vi "cRIO_4DoF_InvYaw_global2mouse_v2.vi"(10 "op-space pos":dbl[](array[numeric]), 11 "op_vel":dbl[](array[numeric])) -> (3 "vel_out":dbl[](array[numeric]))   [LabVIEW 2019]
uses:
  <vilib>/imath/engines/lvmath2/RunTimeEngine/Managers/WorkSpace/UID Generator.vi
  <vilib>/imath/engines/lvmath2/RunTimeEngine/BuiltInFunctions/size/NIMS_[I32,I32]=size(GRow).vi
  <instcachedir>/0/NIMS_[I32,I32]=size(GRow)_CFE2C4BDC5BC45CD88F2F6A295A2273D.lvgen/NIMS_[I32,I32]=size(GRow)_CFE2C4BDC5BC45CD88F2F6A295A2273D_001.vi
  <vilib>/imath/engines/lvmath2/RunTimeEngine/RunTimeType/NIMS_RunTimeType_From StrictType (excl LVString).vi
  <instcachedir>/0/NIMS_RunTimeType_From StrictType (excl LVString)_D8AFBA86A94845AAA577C895450664BD.lvgen/NIMS_RunTimeType_From StrictType (excl LVString)_D8AFBA86A94845AAA577C895450664BD_000.vi
  <vilib>/imath/engines/lvmath2/RunTimeEngine/LocalVariableDefStatement/MC_LocalVariableDefStatement_Display.vi
  <vilib>/imath/engines/lvmath2/RunTimeEngine/IndexRead/NIMS M(R2,S).vi
  <instcachedir>/0/NIMS M(R2,S)_56813DCFDD5A484292D2195AF15D2BF5.lvgen/NIMS M(R2,S)_56813DCFDD5A484292D2195AF15D2BF5_000.vi
  <vilib>/imathl/engines/lvmath/Functions/Error Handling/Create Error.vi
  <vilib>/imath/engines/lvmath2/RunTimeEngine/ArithmeticOperatorToken/NIMS_ArithmeticOperator_multmx(M,CV)-internal.vi
  <instcachedir>/0/NIMS_ArithmeticOperator_multmx(M,CV)-internal_2C55777844884EEDB828A940D397C7D0.lvgen/NIMS_ArithmeticOperator_multmx(M,CV)-internal_2C55777844884EEDB828A940D397C7D0_001.vi
  <vilib>/imath/engines/lvmath2/RunTimeEngine/IndexRead/NIMS M(S,S).vi
  <instcachedir>/0/NIMS M(S,S)_AC51E74150A542F7991B9634C66F3096.lvgen/NIMS M(S,S)_AC51E74150A542F7991B9634C66F3096_000.vi
  <vilib>/imath/engines/lvmath2/RunTimeEngine/Managers/SymbolTable/Clear UID.vi
  <vilib>/imath/engines/lvmath2/RunTimeEngine/NodeEndStatement/NIMS_NodeEndStatement_Output.vi
  <instcachedir>/0/NIMS_NodeEndStatement_Output_53EC0D466D134D7ABD903AC30B43404B.lvgen/NIMS_NodeEndStatement_Output_53EC0D466D134D7ABD903AC30B43404B_005.vi
  <vilib>/imath/engines/lvmath2/RunTimeEngine/ErrorHandling/NIMS_Finalize Error.vi
  <vilib>/imath/engines/lvmath2/RunTimeEngine/Managers/SymbolTable/NIMS_WorkSpace.lvlib
panel:
  out "vel global frame":T1(graph)
  out "vel mouse frame":T1(graph)
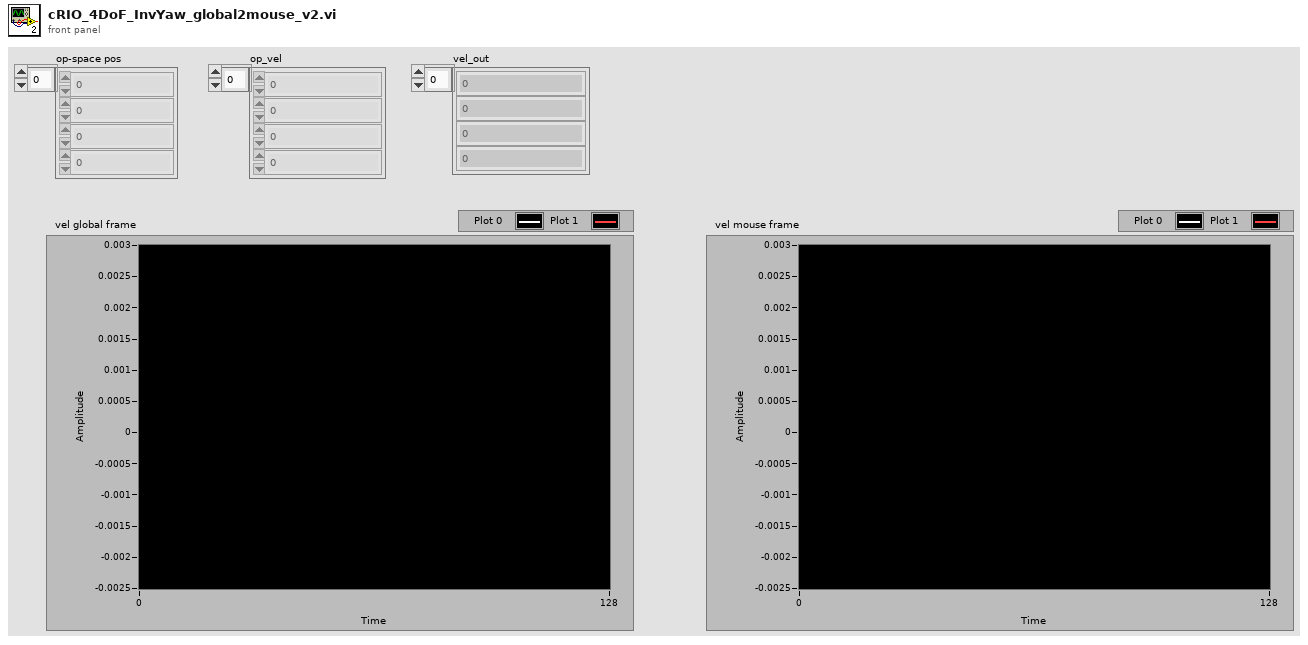
[diagram p1: front panel]
types:
  T1 = cluster{"vel_out[0]":dbl, "vel_out[1]":dbl, "vel_out[2]":dbl, "vel_out[3]":dbl, "vel_out[4]":dbl, "vel_out[5]":dbl, "vel_out[6]":dbl, "vel_out[7]":dbl, "vel_out[8]":dbl}
  T2 = cluster{"op_vel[0]":dbl, "op_vel[1]":dbl, "op_vel[2]":dbl, "op_vel[3]":dbl, "op_vel[4]":dbl, "op_vel[5]":dbl, "op_vel[6]":dbl, "op_vel[7]":dbl, "op_vel[8]":dbl}
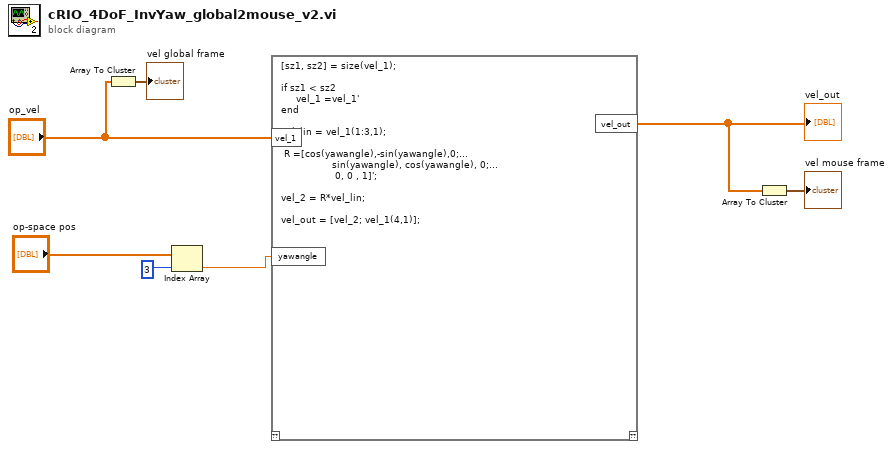
[diagram p0: block diagram]
diagram:
  n1 = Array To Cluster(array="op_vel") -> (cluster=→"vel global frame":T2)
  n2 = Index Array(array="op-space pos", index=3) -> (element=w7:dbl)
  n3 = mathscript code="[sz1, sz2] = size(vel_1);\n\nif sz1 < sz2\n     vel_1 =vel_1'\nend\n\nvel_lin = vel_1(1:3,1);\n\n R =[cos(yawangle),-sin(yawangle),0;...\n                 sin(yawangle), cos(yawangle), 0;...\n                  0, 0 , 1]';\n\nvel_2 = R*vel_lin;\n\nvel_out = [vel_2; vel_1(4,1)];"("vel_1"="op_vel", "yawangle"=w7) -> ("vel_out"=w4:dbl[])  [unwired: 1 in, 1 out]
  "vel_out" <- w4
  n4 = Array To Cluster(array=w4) -> (cluster=→"vel mouse frame":T1)
